vi "Fdx Get Rx UDP Session Status.vi"(8 "error in (no error)":errorcluster, 10 "UdpHandle in":u32, 11 "InstrumentHandle_port in":u32) -> (0 "error out":errorcluster, 1 "MsgCount":u32, 2 "UdpHandle out":u32, 3 "InstrumentHandle_port out":u32, 4 "MsgErrorCount":u32)   [LabVIEW 2020, in "AIM664LV.lvlib"]
uses:
  AIM664LV.lvlib
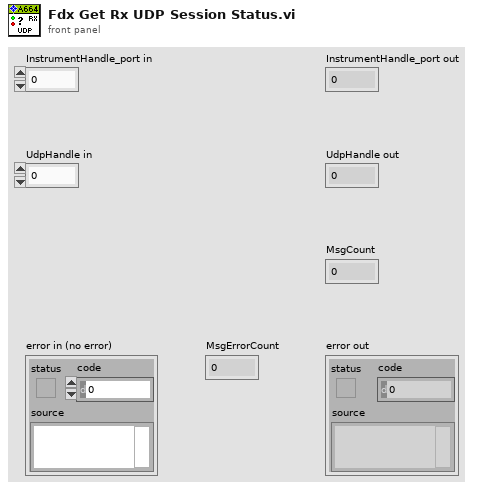
[diagram p1: front panel]
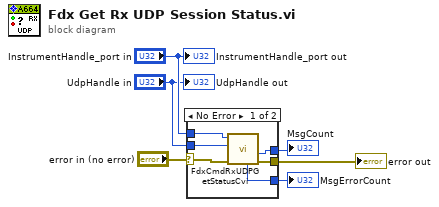
[diagram p0: block diagram]
diagram:
  n1 = case shown="No Error" "error in (no error)" {
    selector: "error in (no error)" -> [w12 w13]
    tunnel: [w11 w13] -> w5
    tunnel: [w10 _] -> w1
    tunnel: "InstrumentHandle_port in" -> [w9 _]
    tunnel: "UdpHandle in" -> [w8 _]
    tunnel: [w7 _] -> w2
    frame No Error {
      n2 = call "FdxCmdRxUDPGetStatusCvi.vi"("error in"=w12, "UdpHandle"=w8, "InstrumentHandle_port"=w9) -> ("error out"=w11:errorcluster, "MsgCount"=w10:u32, "MsgErrorCount"=w7:u32)  [unwired: 4 in, 2 out]
    }
    frame Error {
    }
  }
  "error out" <- w5
  "MsgErrorCount" <- w2
  "MsgCount" <- w1
  "InstrumentHandle_port out" <- "InstrumentHandle_port in"
  "UdpHandle out" <- "UdpHandle in"
